vi "EMS Measurement Visualization.vi"(4 "Measurement/Error":string, 8 "error in (no error)":errorcluster, 9 "Measurement Name":string, 10 "IED Name":string, 11 "Master Controller in":refnum<class "Master Controller.lvclass">) -> (0 "error out":errorcluster, 3 "Master Controller out":refnum<class "Master Controller.lvclass">)   [LabVIEW 2015, in "Master Controller Core.lvlib" / "Master Controller.lvclass"]
uses:
  Master Controller.lvclass
  Communications/SCADA Communcations Actor/SCADA Communications/Controls/EMS Message Cluster.ctl
  Master Controller.lvclass/Master Controller.ctl
  Communications/SCADA Communcations Actor/SCADA Communications Messages/Transmit EMS Message Msg/Transmit EMS Message Msg.lvclass/Transmit EMS Message Msg.ctl
  <vilib>/ActorFramework/Message Enqueuer/Message Enqueuer.lvclass/Message Enqueuer.ctl
  <vilib>/ActorFramework/Message Enqueuer/Enqueue.vi
  <vilib>/ActorFramework/Message Priority Queue/Priority Enqueue.vi
  Communications/SCADA Communcations Actor/SCADA Communications Messages/Transmit EMS Message Msg/Transmit EMS Message Msg.lvclass
  Utilities/Message Strings.llb/Message String Utilities.lvlib
  Communications/SCADA Communcations Actor/SCADA Communications/SCADA Communications.lvclass
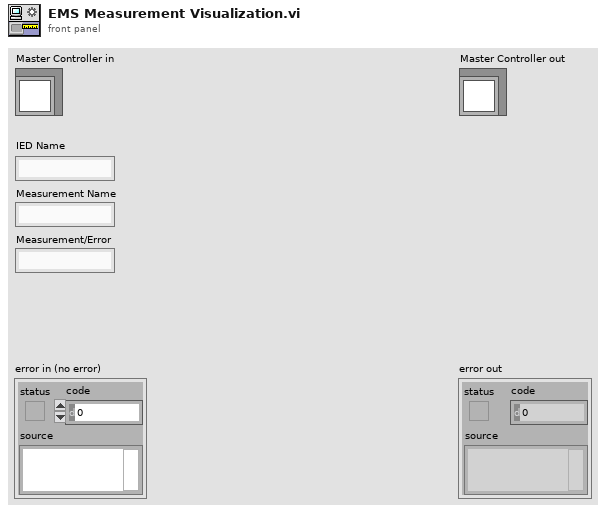
[diagram p1: front panel]
types:
  T1 = typedef "SCADA Communcations Actor.lvlib/SCADA Communications.lvclass/EMS Message Cluster.ctl" = cluster{"Name":string, "Content":string}
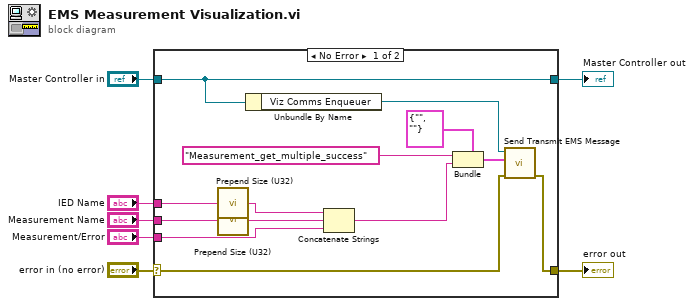
[diagram p0: block diagram]
diagram:
  n1 = case shown="No Error" "error in (no error)" {
    selector: "error in (no error)" -> [w15 w22]
    tunnel: [w14 w22] -> w6
    tunnel: [w16 w21] -> w4
    tunnel: "Master Controller in" -> [w16 w21]
    tunnel: "IED Name" -> [w13 _]
    tunnel: "Measurement Name" -> [w12 _]
    tunnel: "Measurement/Error" -> [w11 _]
    frame No Error {
      n2 = call "Prepend Size (U32).vi"("String in"=w13) -> ("String out"=w8:string)
      n3 = call "Prepend Size (U32).vi"("String in"=w12) -> ("String out"=w9:string)
      n4 = Unbundle By Name(w16) -> ("Viz Comms Enqueuer"=w18:refnum<class "Message Enqueuer.lvclass">)
      n5 = Concatenate Strings(w8, w9, w11) -> (w10:string)
      n6 = Bundle(cluster=T1 {"Name"="", "Content"=""} ("Message"), "Name"="Measurement_get_multiple_success", "Content"=w10) -> (w19:T1)
      n7 = call "Send Transmit EMS Message.vi"("error in (no error)"=w15, "Message"=w19, "Message Enqueuer"=w18) -> ("error out"=w14:errorcluster)  [unwired: 7 in, 1 out]
    }
    frame Error {
    }
  }
  "error out" <- w6
  "Master Controller out" <- w4
